vi "main.vi"() -> ()   [LabVIEW 2018]
doc: "This example demonstrates the use of binary morphological reconstruction in the particle analysis. The example allows you to keep the particles completely inside the ROI, completely outside the ROI or on the ROI."
uses:
  <vilib>/vision/NI_Vision_Development_Module.lvlib
panel:
  in  "条件1-面积判断":T2(array[cluster]) {"Measurement Parameter" items=["Area"]; "下限" format="%.2f"; "上限" format="%.2f"}
  in  "条件2-灰度阈值":cluster{"下限":sgl, "上限":sgl}={"下限"=128.0, "上限"=255.0} {"下限" min=0 max=255 step=1; "上限" min=0 max=255 step=1}
  in  "查看标注":bool
  in  "最终报告":bool
  in  "导入图像":bool
  in  "删除标注":bool
  in  "退出":bool
  out "标注框总数":dbl
  out "全图灰度级信息":T3 {"标准差" format="%.2f"; "均值" format="%.2f"; "相邻灰度级间隔" format="%.2f"; "起始灰度值" format="%.2f"; "最大值" format="%.2f"; "最小值" format="%.2f"}
  out "全图灰度表":u32[](graph)
  in  "Font, Size & Style 2":T4={"Desired Font (Application)"=enum."Application Font", "[User-specified Font]"={"Font Name"="", "Size"=12, "Strikeout?"=FALSE, "Italic?"=FALSE, "Underline?"=FALSE, "Outline?"=FALSE, "Shadow?"=FALSE, "Bold?"=FALSE, "Rotation Angle"=0.0}, "Horizontal Alignment"=0, "Vertical Alignment"=0} {"Vertical Alignment" items=["Bottom", "Top", "Baseline"]; "Horizontal Alignment" items=["Left", "Center", "Right"]; "[User-specified Font]"."Rotation Angle" format="%.2f"}
  in  "Font, Size & Style":T4={"Desired Font (Application)"=enum."Application Font", "[User-specified Font]"={"Font Name"="", "Size"=12, "Strikeout?"=FALSE, "Italic?"=FALSE, "Underline?"=FALSE, "Outline?"=FALSE, "Shadow?"=FALSE, "Bold?"=FALSE, "Rotation Angle"=0.0}, "Horizontal Alignment"=0, "Vertical Alignment"=0} {"Vertical Alignment" items=["Bottom", "Top", "Baseline"]; "Horizontal Alignment" items=["Left", "Center", "Right"]; "[User-specified Font]"."Rotation Angle" format="%.2f"}
  out "框组":T5(array[cluster])
  in  "Operation":enum16{"overlay rectangle"}(ring)
  out "标注图":T6(plugin-control)
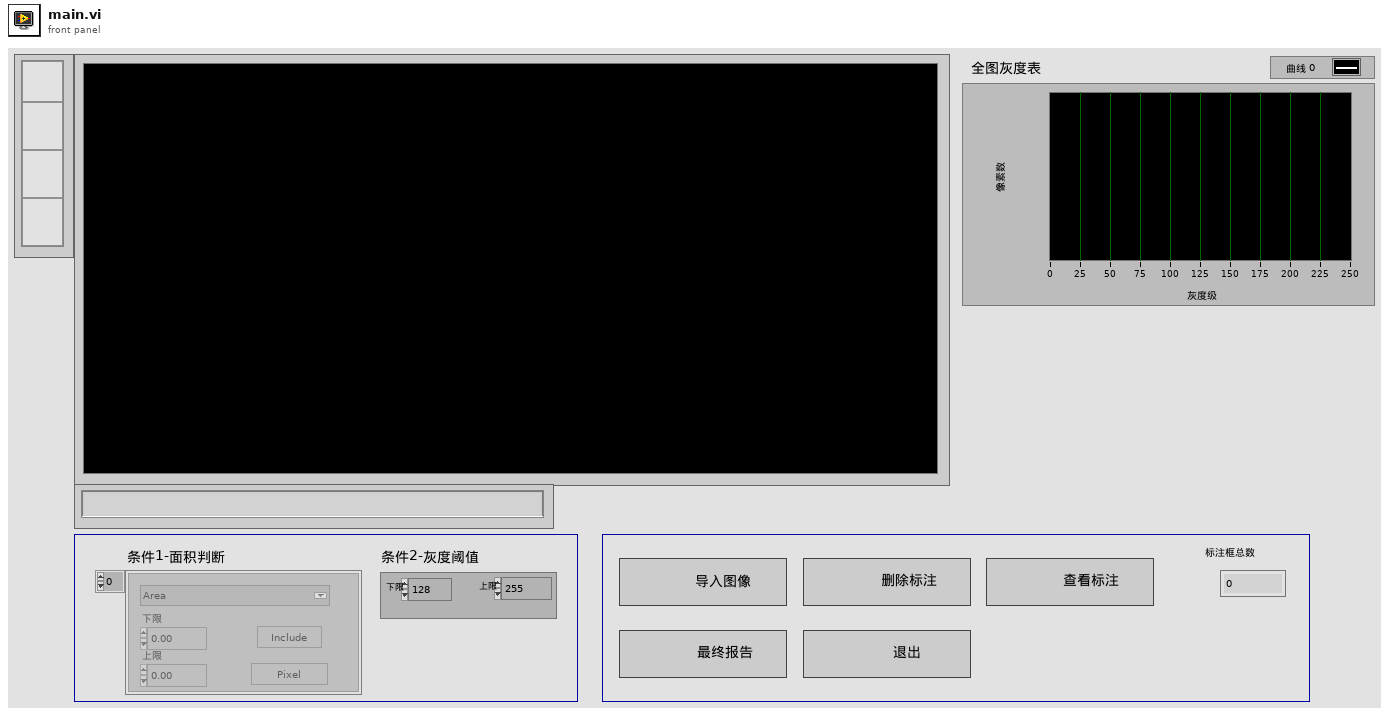
[diagram p1: front panel]
types:
  T1 = typedef "Particle Parameters" = i32
  T2 = cluster{"Measurement Parameter":T1, "下限":dbl, "上限":dbl, "Range":bool, "Measurement Type":bool}[]
  T3 = cluster{"histogram":u32[], "最小值":sgl, "最大值":sgl, "起始灰度值":sgl, "相邻灰度级间隔":sgl, "均值":sgl, "标准差":sgl, "像素面积":i32}
  T4 = cluster{"Desired Font (Application)":enum16{"User-specified Font", "Application Font", "System Font", "Dialog Font"}, "[User-specified Font]":cluster{"Font Name":string, "Size":i16, "Strikeout?":bool, "Italic?":bool, "Underline?":bool, "Outline?":bool, "Shadow?":bool, "Bold?":bool, "Rotation Angle":dbl}, "Horizontal Alignment":i16, "Vertical Alignment":i16}
  T5 = cluster{"Global Rectangle":i32[], "Contours":cluster{"Contour Type":u32, "ROI Type":u32, "Points":i32[]}[]}[]
  T6 = typedef "IMAQ Image.ctl" = refnum<image>
  T7 = typedef "Image Type" = u32
  T8 = cluster{"Global Rectangle":i32[], "Contours":cluster{"Contour Type":u32, "ROI Type":u32, "Points":i32[]}[]}
  T9 = cluster{"histogram":u32[], "Minimal Value":sgl, "Maximal Value":sgl, "Starting Value":sgl, "Interval Width":sgl, "Mean Value":sgl, "Standard  Variation":sgl, "Area (pixels)":i32}
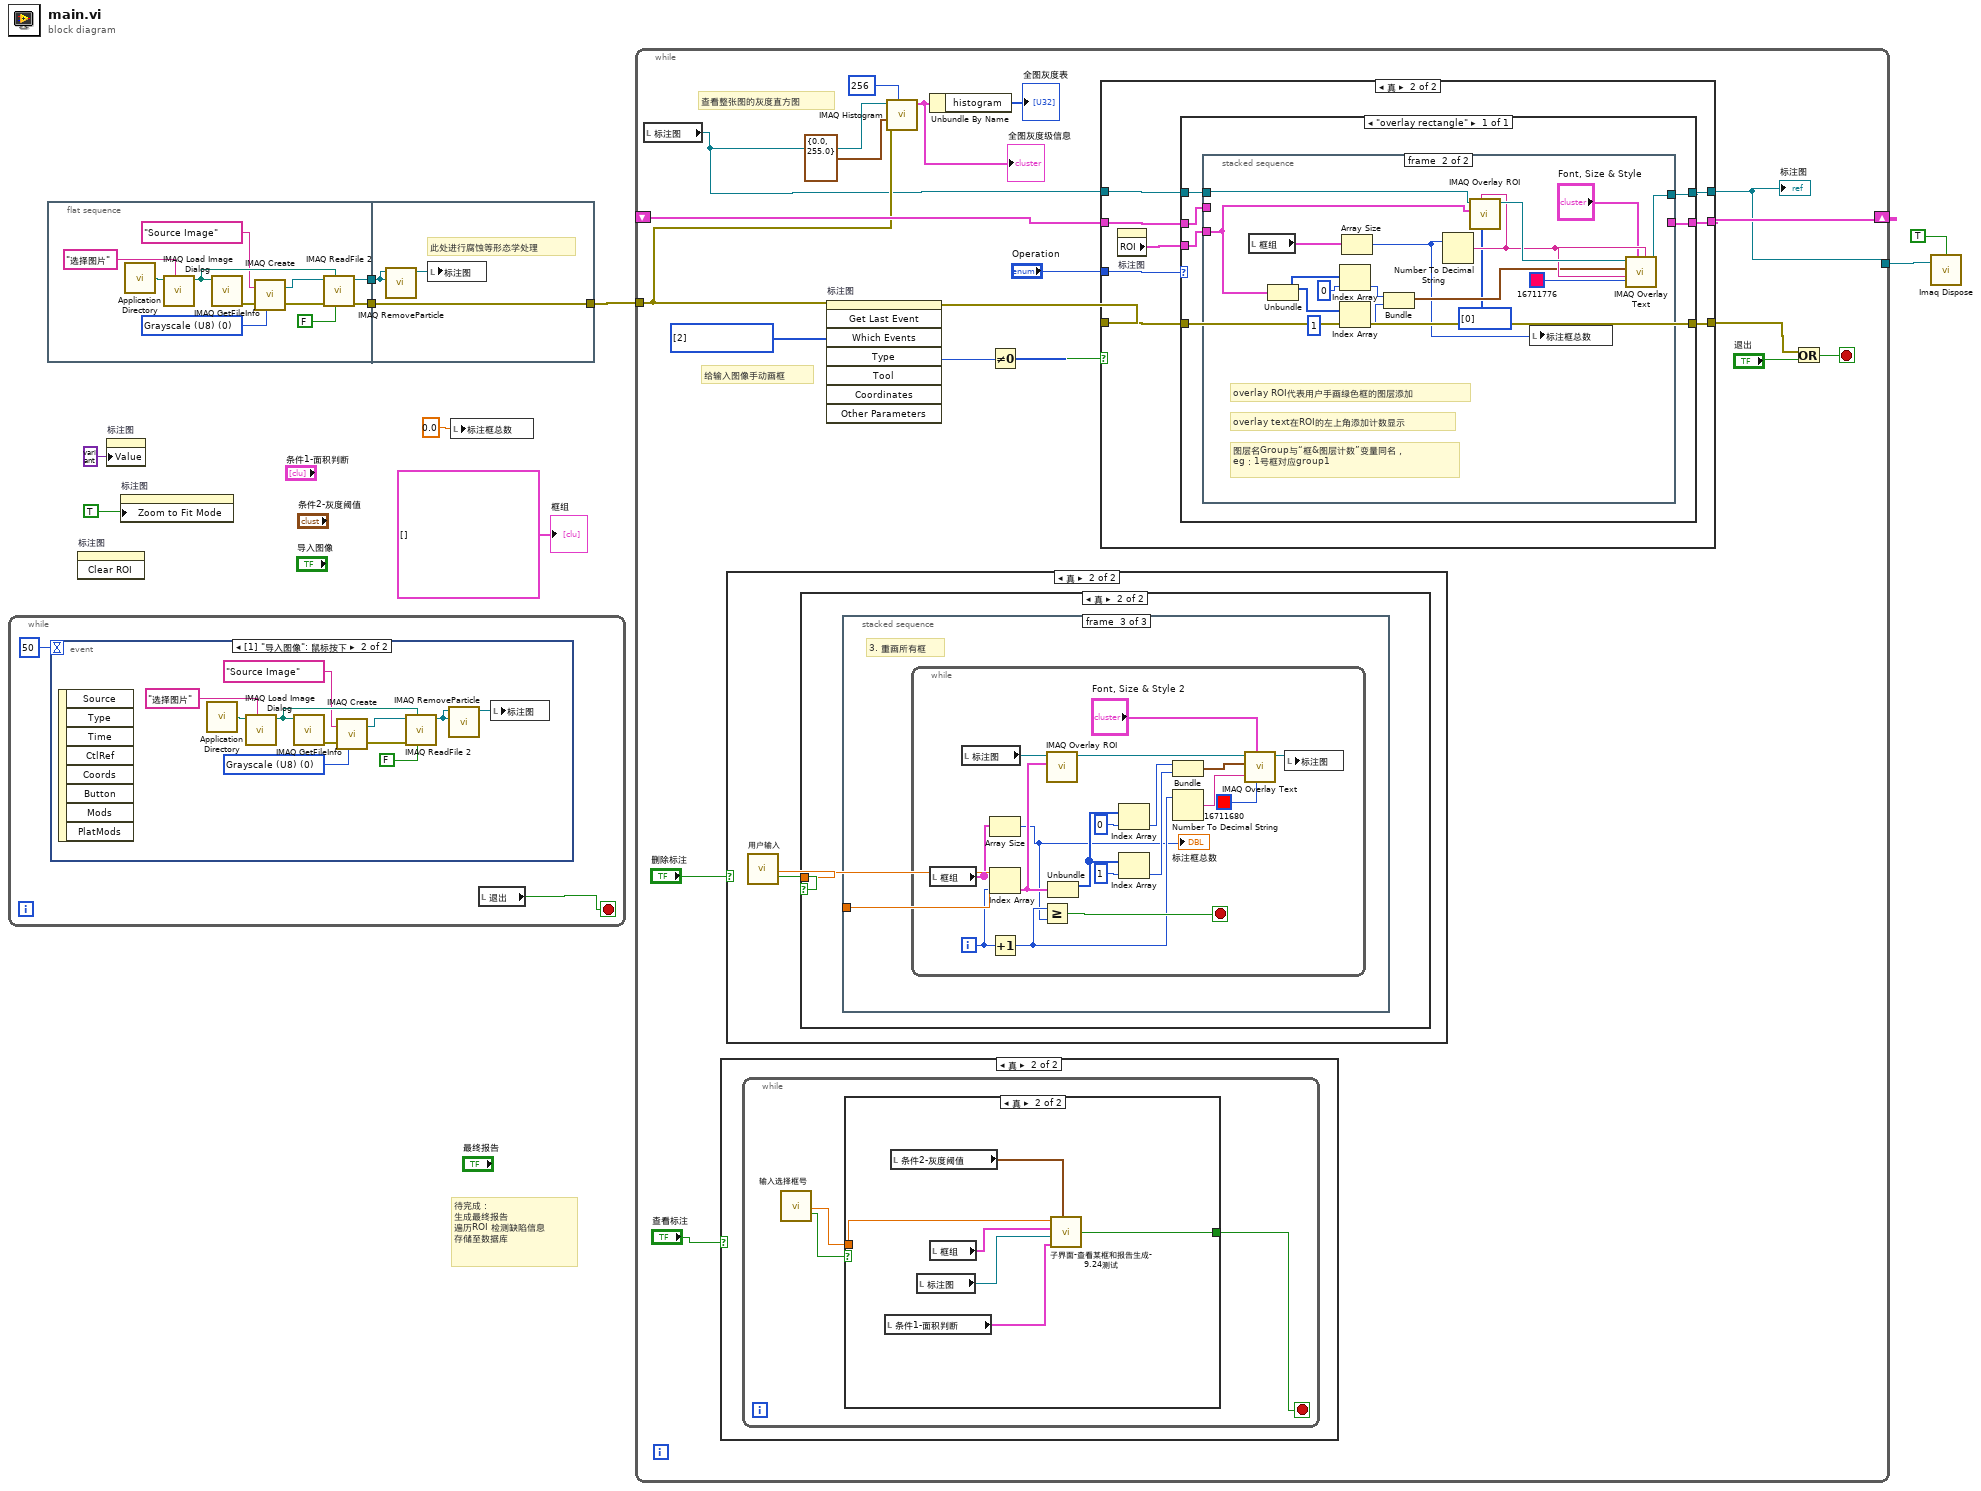
[diagram p0: block diagram]
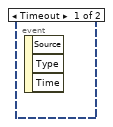
[diagram p2: hidden frame]
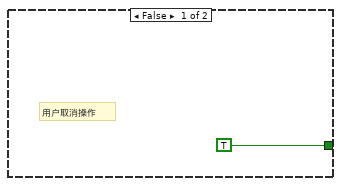
[diagram p4: hidden frame]
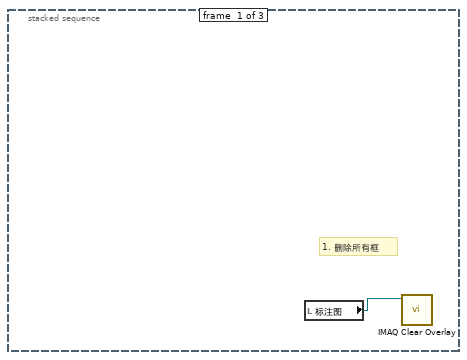
[diagram p7: hidden frame]
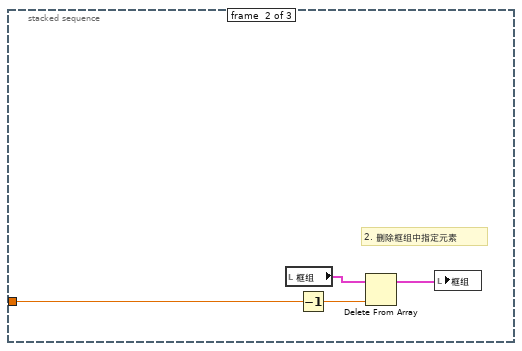
[diagram p8: hidden frame]
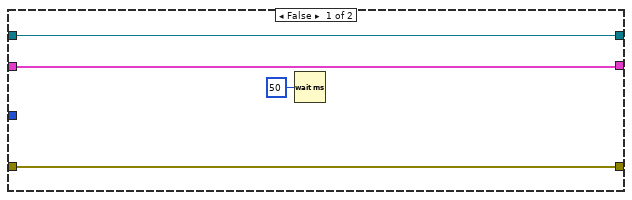
[diagram p9: hidden frame]
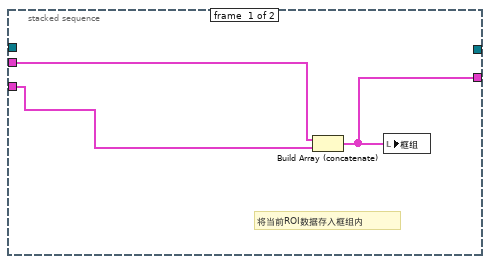
[diagram p10: hidden frame]
diagram:
  # "待完成：\n生成最终报告\n遍历ROI 检测缺陷信息\n存储至数据库"
  n1 = while {
    stop <- w10 stop-if-true
    n2 = event shown="[1] \"导入图像\": 鼠标按下" {
      selector: _ -> [_ _]
      dyn-events: _ -> [_ _]
      timeout: 50 -> [_ _]
      event Timeout {
        n3 = event-data() -> ()  [unwired: 1 in, 3 out]
      }
      event "导入图像": Mouse Down {
        w14 = T7 0 items=["Grayscale (U8)", "Grayscale (I16)", "Grayscale (SGL)", "Complex (CSG)", "RGB (U32)", "HSL (U32)", "RGB (U64)", "Grayscale (U16)"] ("Image Type")
        n4 = event-data() -> ()  [unwired: 1 in, 8 out]
        n5 = call <vilib>:"Application Directory.vi"() -> ("Application Directory"=w22:path)
        n6 = call "IMAQ Load Image Dialog"("Prompt"="选择图片" ("prompt"), "Start Path"=w22) -> ("Path"=w18:path)  [unwired: 7 in, 2 out]
        n7 = call "IMAQ GetFileInfo"("File Path"=w18) -> ("error out"=w19:errorcluster)  [unwired: 4 in, 6 out]
        n8 = call "IMAQ Create"("Image Name"="Source Image", "Image Type"=w14, "error in (no error)"=w19) -> ("New Image"=w20:T6, "error out"=w21:errorcluster)  [unwired: 2 in]
        n9 = call "IMAQ ReadFile 2"("Use File Path Image Type"=FALSE, "File Path"=w18, "error in (no error)"=w21, "Image"=w20) -> ("Image Out"=w13:T6)  [unwired: 3 in, 4 out]
        n10 = call "IMAQ RemoveParticle"("Image Dst"=w13, "Image Src"=w13) -> ("Image Dst Out"=w12:T6)  [unwired: 8 in, 1 out]
        n11 = local write "标注图"(w12) -> ()
      }
    }
    n12 = local read "退出"() -> (w10:bool)
  }
  n13 = flat-sequence {
    tunnel: [w24] -> w2
    tunnel: [w23] -> w1
    tunnel: [w36] -> w9
    tunnel: w2 -> [w36]
    tunnel: w1 -> [w35]
    frame #0 {
      w25 = T7 0 items=["Grayscale (U8)", "Grayscale (I16)", "Grayscale (SGL)", "Complex (CSG)", "RGB (U32)", "HSL (U32)", "RGB (U64)", "Grayscale (U16)"] ("Image Type")
      n14 = call <vilib>:"Application Directory.vi"() -> ("Application Directory"=w33:path)
      n15 = call "IMAQ Load Image Dialog"("Prompt"="选择图片" ("prompt"), "Start Path"=w33) -> ("Path"=w29:path)  [unwired: 7 in, 2 out]
      n16 = call "IMAQ GetFileInfo"("File Path"=w29) -> ("error out"=w30:errorcluster)  [unwired: 4 in, 6 out]
      n17 = call "IMAQ Create"("Image Name"="Source Image", "Image Type"=w25, "error in (no error)"=w30) -> ("New Image"=w31:T6, "error out"=w32:errorcluster)  [unwired: 2 in]
      n18 = call "IMAQ ReadFile 2"("Use File Path Image Type"=FALSE, "File Path"=w29, "error in (no error)"=w32, "Image"=w31) -> ("error out"=w24:errorcluster, "Image Out"=w23:T6)  [unwired: 3 in, 3 out]
    }
    frame #1 {
      # "此处进行腐蚀等形态学处理"
      n19 = call "IMAQ RemoveParticle"("Image Dst"=w35, "Image Src"=w35) -> ("Image Dst Out"=w34:T6)  [unwired: 8 in, 1 out]
      n20 = local write "标注图"(w34) -> ()
    }
  }
  n21 = invoke on="标注图" class="ImageControl" method="Clear ROI"() -> ()  [unwired: 3 in, 3 out]
  n22 = property on="标注图" class="ImageControl"("Value"=variant ("值")) -> ()  [unwired: 2 in, 2 out]
  n23 = property on="标注图" class="ImageControl"("Zoom to Fit Mode"=TRUE) -> ()  [unwired: 2 in, 2 out]
  n24 = local write "标注框总数"(0.0 ("框总数")) -> ()
  n25 = while {
    shift-right: [w48] -> _
    shift-left: _ -> [w47]
    tunnel: w9 -> [w46]
    tunnel: [w38] -> w4
    stop <- w50 stop-if-true
    w53 = i32[] [2] items=["No Event"=0, "Click Event"=1, "Draw Event"=2, "Size Event"=4, "Scroll Event"=5, "Double Click Event"=8] ("Which Events")
    # "给输入图像手动画框"
    # "查看整张图的灰度直方图"
    n26 = local read "标注图"() -> (w39:T6)
    n27 = case shown="真" "查看标注" {
      frame False {
      }
      frame True {
        n28 = while {
          stop <- w56 stop-if-true
          n29 = call "输入选择框号"() -> ("框号"=w58:dbl, "确定"=w57:bool)  [unwired: 17 in, 1 out]
          n30 = case shown="真" w57 {
            tunnel: w58 -> [_ w65]
            tunnel: [TRUE ("返回 2") w60] -> w56
            frame False {
              # "用户取消操作"
            }
            frame True {
              n31 = local read "条件1-面积判断"() -> (w61:T2)
              n32 = local read "条件2-灰度阈值"() -> (w62:cluster{"下限":sgl, "上限":sgl})
              n33 = local read "标注图"() -> (w63:T6)
              n34 = local read "框组"() -> (w64:T5)
              n35 = call "子界面-查看某框和报告生成-9.24测试.vi"("框号"=w65, "框组"=w64, "标注图"=w63, "条件1-面积判断"=w61, "条件2-灰度阈值"=w62) -> ("返回 2"=w60:bool)
            }
          }
        }
      }
    }
    n36 = case shown="真" "删除标注" {
      frame False {
      }
      frame True {
        n37 = call "用户输入"() -> ("框号"=w66:dbl, "确定"=w67:bool)  [unwired: 17 in, 1 out]
        n38 = case shown="真" w67 {
          tunnel: w66 -> [_ w68]
          frame False {
            # "用户取消操作"
          }
          frame True {
            n39 = stacked-sequence {
              tunnel: w68 -> [_ w72 _]
              frame #0 {
                # "1. 删除所有框"
                n40 = local read "标注图"() -> (w69:T6)
                n41 = call "IMAQ Clear Overlay"("Image"=w69) -> ()  [unwired: 9 in, 2 out]
              }
              frame #1 {
                # "2. 删除框组中指定元素"
                n42 = local read "框组"() -> (w73:T5)
                n43 = Decrement(x=w72) -> (x-1=w71:dbl)
                n44 = Delete From Array(array=w73, index=w71) -> (array with subset deleted=w70:T5)  [unwired: 1 in, 1 out]
                n45 = local write "框组"(w70) -> ()
              }
              frame #2 {
                # "3. 重画所有框"
                n46 = while {
                  i -> [w76]
                  stop <- w91 stop-if-true
                  n47 = local read "框组"() -> (w84:T5)
                  n48 = local read "标注图"() -> (w90:T6)
                  n49 = Array Size(array=w84) -> (size(s)=w74:i32)
                  "标注框总数" <- w74
                  n50 = Index Array(array=w84, index=w76) -> (element=w77:T8)
                  n51 = Increment(x=w76) -> (x+1=w89:i32)
                  n52 = Greater Or Equal?(x=w89, y=w74) -> (x >= y?=w91:bool)
                  n53 = call "IMAQ Overlay ROI"("ROI Descriptor"=w77, "Image"=w90) -> ("Image Out"=w86:T6)  [unwired: 8 in, 1 out]
                  n54 = Unbundle(w77) -> ("Global Rectangle"=w80:i32[])  [unwired: 1 out]
                  n55 = Index Array(array=w80, index=0 ("索引")) -> (element=w81:i32)
                  n56 = Index Array(array=w80, index=1 ("索引")) -> (element=w82:i32)
                  n57 = Bundle(w81, w82) -> (w79:cluster{i32, i32})  [unwired: 1 in]
                  n58 = Number To Decimal String(number=w89) -> (decimal integer string=w87:string)  [unwired: 1 in]
                  n59 = call "IMAQ Overlay Text"("Text Color (black)"=u32 16711680, "Font, Size & Style"="Font, Size & Style 2", "String"=w87, "Origin"=w79, "Image"=w86) -> ("Image Out"=w85:T6)  [unwired: 5 in, 1 out]
                  n60 = local write "标注图"(w85) -> ()
                }
              }
            }
          }
        }
      }
    }
    n61 = invoke on="标注图" class="ImageControl" method="Get Last Event"(error in=w46, "Which Events"=w53) -> (error out=w52:errorcluster, "Type"=w54:i32)  [unwired: 6 in, 6 out]
    n62 = call "IMAQ Histogram"("Number of Classes"=256, "error in (no error)"=w46, "Interval Range"=cluster{"Minimum":sgl, "Maximum":sgl} {"Minimum"=0.0, "Maximum"=255.0}, "Image"=w39) -> ("Histogram Report"=w43:T9)  [unwired: 6 in, 1 out]
    "全图灰度级信息" <- w43
    n63 = Unbundle By Name(w43) -> ("histogram"=→"全图灰度表":u32[])
    n64 = Not Equal To 0?(x=w54) -> (x != 0?=w49:bool)
    n65 = case shown="真" w49 {
      tunnel: w39 -> [w95 w103]
      tunnel: [w95 w102] -> w38
      tunnel: "Operation" -> [_ w100]
      tunnel: w52 -> [w94 w99]
      tunnel: [w94 w98] -> w51
      tunnel: [w92 w97] -> w48
      tunnel: w47 -> [w92 w96]
      frame False {
        n66 = Wait (ms)(milliseconds to wait=u32 50) -> ()  [unwired: 1 out]
      }
      frame True {
        n67 = property on="标注图" class="ImageControl"() -> ("ROI"=w101:T8)  [unwired: 2 in, 2 out]
        n68 = case shown="\"overlay rectangle\"" w100 {
          tunnel: w103 -> [w108]
          tunnel: w101 -> [w106]
          tunnel: [w107] -> w102
          tunnel: w99 -> [w109]
          tunnel: [w109] -> w98
          tunnel: [w105] -> w97
          tunnel: w96 -> [w104]
          frame "overlay rectangle" {
            n69 = stacked-sequence {
              tunnel: w108 -> [_ w119]
              tunnel: [_ w118] -> w107
              tunnel: w106 -> [w112 w115]
              tunnel: [w110 _] -> w105
              tunnel: w104 -> [w111 _]
              frame #0 {
                # "将当前ROI数据存入框组内"
                n70 = Build Array (concatenate)(w111, w112) -> (w110:T5)
                n71 = local write "框组"(w110) -> ()
              }
              frame #1 {
                # "图层名Group与“框&图层计数”变量同名，\neg：1号框对应group1"
                # "overlay text在ROI的左上角添加计数显示"
                # "overlay ROI代表用户手画绿色框的图层添加"
                n72 = local read "框组"() -> (w124:T5)
                n73 = Unbundle(w115) -> ("Global Rectangle"=w127:i32[])  [unwired: 1 out]
                n74 = Index Array(array=w127, index=0 ("索引")) -> (element=w126:i32)
                n75 = Index Array(array=w127, index=1 ("索引")) -> (element=w125:i32)
                n76 = Array Size(array=w124) -> (size(s)=w113:i32)
                n77 = Bundle(w126, w125) -> (w117:cluster{i32, i32})  [unwired: 1 in]
                n78 = Number To Decimal String(number=w113) -> (decimal integer string=w123:string)  [unwired: 1 in]
                n79 = call "IMAQ Overlay ROI"("Colors (Green)"=u32[] [0], "Group"=w123, "ROI Descriptor"=w115, "Image"=w119) -> ("Image Out"=w128:T6)  [unwired: 6 in, 1 out]
                n80 = local write "标注框总数"(w113) -> ()
                n81 = call "IMAQ Overlay Text"("Group"=w123, "Text Color (black)"=u32 16711776, "Font, Size & Style"="Font, Size & Style", "String"=w123, "Origin"=w117, "Image"=w128) -> ("Image Out"=w118:T6)  [unwired: 4 in, 1 out]
              }
            }
          }
        }
      }
    }
    "标注图" <- w38
    n82 = Or(x=w51, y="退出") -> (x .or. y?=w50:bool)
  }
  n83 = call "Imaq Dispose"("All Images? (No)"=TRUE, "Image"=w4) -> ()  [unwired: 1 in, 4 out]
  "框组" <- T5 [] ("框组")
